vi "Lock SPAN Registers.vi"(11 "active SPAN Index":i32) -> (3 "Array":string[](array[string]))   [LabVIEW 2020, in "Linearisierung v2.lvlib" / "SpanEinstellungen.lvlib"]
uses:
  SpanEinstellungen.lvlib
  Aktion FGV SpanEinstellungen.ctl
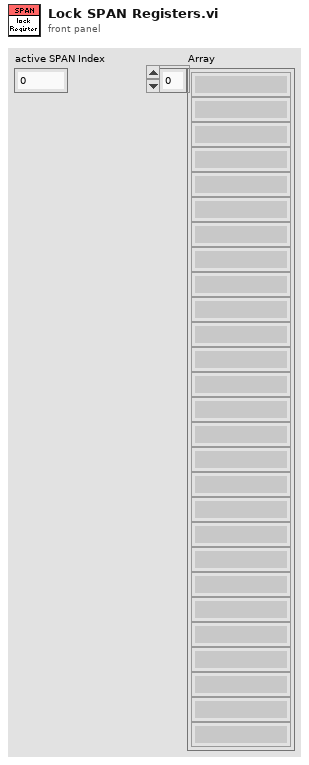
[diagram p1: front panel]
types:
  T1 = typedef "Linearisierung v2.lvlib/SpanEinstellungen.lvlib/Aktion FGV SpanEinstellungen.ctl" = enum16{"lesen", "schreiben", "laden", "speichern", "RegisterRef", "automatisch", "init", "PDF Params", "Punkte umkehren"}
  T2 = cluster{"HauptRegister in":refnum<vi>, "SpanRegister in":refnum<vi>}
  T3 = enum8{"Enabled", "Disabled", "Disabled and Grayed Out"}
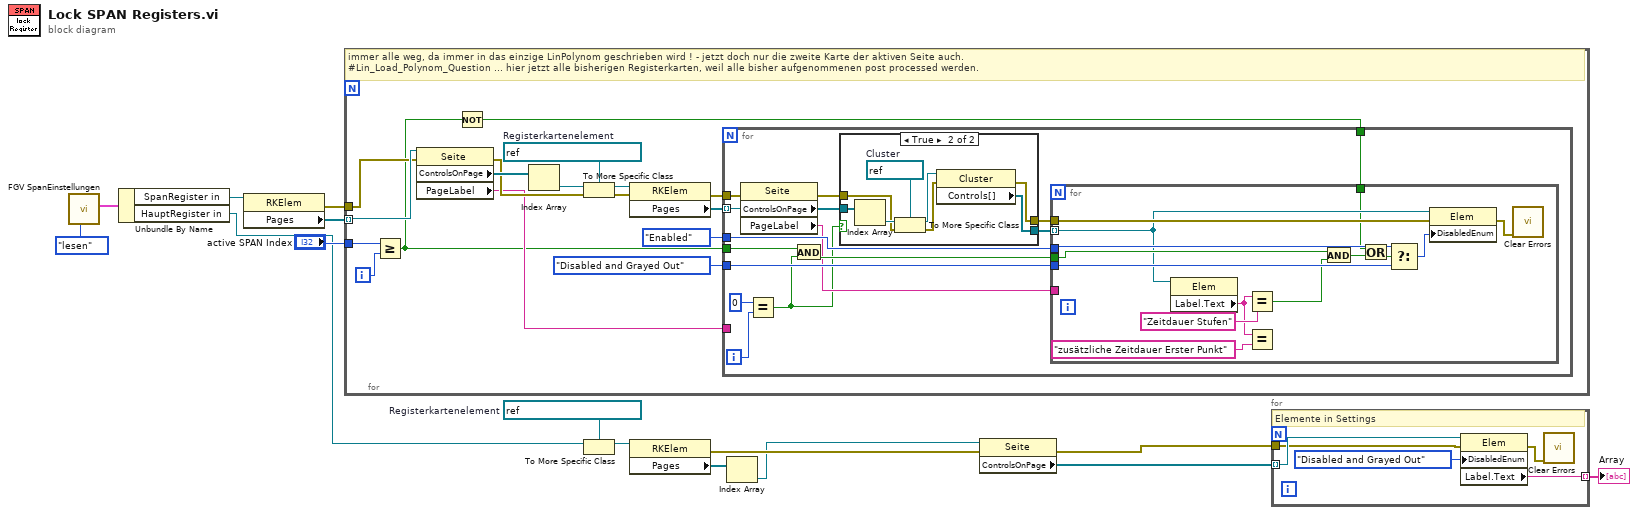
[diagram p0: block diagram]
diagram:
  w10 = refnum<vi> refnum  # Registerkartenelement
  n1 = call "FGV SpanEinstellungen.vi"("Aktion"=Aktion_FGV_SpanEinstellungen."lesen") -> ("RegisterRefs out"=w15:T2)  [unwired: 6 in, 4 out]
  n2 = Unbundle By Name(w15) -> ("SpanRegister in"=w3:refnum<vi>, "HauptRegister in"=w2:refnum<vi>)
  n3 = property class="RKElem"(reference=w3) -> (error out=w11:errorcluster, "Pages"=w12:refnum<vi>[])  [unwired: 1 in, 1 out]
  n4 = for {
    tunnel: w12 -> [w32] mode=indexing
    tunnel: w11 -> [w23]
    tunnel: "active SPAN Index" -> [w21]
    i -> [w22]
    w29 = refnum<vi> refnum  # Registerkartenelement
    # "immer alle weg, da immer in das einzige LinPolynom geschrieben wird ! - jetzt doch nur die zweite Karte der aktiven Seite auch.\n#Lin_Load_Polynom_Question ... hier jetzt alle bisherigen Registerkarten, weil alle bisher aufgenommenen post processed werden."
    n5 = Greater Or Equal?(x=w21, y=w22) -> (x >= y?=w17:bool)
    n6 = property class="Seite"(reference=w32, error in=w23) -> (error out=w26:errorcluster, "ControlsOnPage"=w31:refnum<vi>[], "PageLabel"=w20:string)  [unwired: 1 out]
    n7 = Not(x=w17) -> (.not. x?=w16:bool)
    n8 = Index Array(array=w31) -> (element=w30:refnum<vi>)  [unwired: 1 in]
    n9 = To More Specific Class(target class=w29, reference=w30, error in=w26) -> (specific class reference=w28:refnum<vi>, error out=w27:errorcluster)
    n10 = property class="RKElem"(reference=w28, error in=w27) -> (error out=w24:errorcluster, "Pages"=w25:refnum<vi>[])  [unwired: 1 out]
    n11 = for {
      tunnel: w25 -> [w47] mode=indexing
      tunnel: w24 -> [w46]
      tunnel: T3."Disabled and Grayed Out" ("Deaktiviert") -> [w42]
      tunnel: T3."Enabled" ("Deaktiviert") -> [w40]
      tunnel: w17 -> [w45]
      tunnel: w20 -> [_]
      tunnel: w16 -> [w33]
      i -> [w44]
      n12 = property class="Seite"(reference=w47, error in=w46) -> (error out=w38:errorcluster, "ControlsOnPage"=w36:refnum<vi>[], "PageLabel"=w39:string)  [unwired: 1 out]
      n13 = Equal?(x=0, y=w44) -> (x = y?=w35:bool)
      n14 = And(x=w45, y=w35) -> (x .and. y?=w41:bool)
      n15 = case shown="True" w35 {
        tunnel: w38 -> [w48 w54]
        tunnel: [w48 w57] -> w37
        tunnel: w36 -> [w49 w56]
        tunnel: [w49 w50] -> w34
        frame False {
        }
        frame True {
          w52 = refnum<vi> refnum  # Cluster
          n16 = Index Array(array=w56) -> (element=w55:refnum<vi>)  [unwired: 1 in]
          n17 = To More Specific Class(target class=w52, reference=w55, error in=w54) -> (specific class reference=w51:refnum<vi>, error out=w53:errorcluster)
          n18 = property class="Cluster"(reference=w51, error in=w53) -> (error out=w57:errorcluster, "Controls[]"=w50:refnum<vi>[])  [unwired: 1 out]
        }
      }
      n19 = for {
        tunnel: w34 -> [w64] mode=indexing
        tunnel: w37 -> [w71]
        tunnel: w42 -> [w69]
        tunnel: w41 -> [w68]
        tunnel: w40 -> [w67]
        tunnel: w39 -> [_]
        tunnel: w33 -> [w58]
        n20 = property class="Elem"(reference=w64) -> ("Label.Text"=w61:string)  [unwired: 1 in, 2 out]
        n21 = Equal?(x=w61, y="Zeitdauer Stufen") -> (x = y?=w63:bool)
        n22 = Equal?(x=w61, y="zusätzliche Zeitdauer Erster Punkt") -> ()  [unwired: 1 out]
        n23 = And(x=w68, y=w63) -> (x .and. y?=w65:bool)
        n24 = Or(x=w58, y=w65) -> (x .or. y?=w59:bool)
        n25 = Select(t=w67, s=w59, f=w69) -> (s? t:f=w66:T3)
        n26 = property class="Elem"(reference=w64, error in=w71, "DisabledEnum"=w66) -> (error out=w70:errorcluster)  [unwired: 1 out]
        n27 = call <vilib>:"Clear Errors.vi"("error in (no error)"=w70) -> ()  [unwired: 5 in, 2 out]
      }
    }
  }
  n28 = To More Specific Class(target class=w10, reference=w2) -> (specific class reference=w9:refnum<vi>)  [unwired: 1 in, 1 out]
  n29 = property class="RKElem"(reference=w9) -> (error out=w8:errorcluster, "Pages"=w7:refnum<vi>[])  [unwired: 1 in, 1 out]
  n30 = Index Array(array=w7) -> (element=w6:refnum<vi>)  [unwired: 1 in]
  n31 = property class="Seite"(reference=w6, error in=w8) -> (error out=w4:errorcluster, "ControlsOnPage"=w5:refnum<vi>[])  [unwired: 1 out]
  n32 = for {
    tunnel: w5 -> [w76] mode=indexing
    tunnel: w4 -> [w74]
    tunnel: [w72] -> w1 mode=indexing
    # "Elemente in Settings"
    n33 = property class="Elem"(reference=w76, error in=w74, "DisabledEnum"=T3."Disabled and Grayed Out" ("Deaktiviert")) -> (error out=w73:errorcluster, "Label.Text"=w72:string)  [unwired: 1 out]
    n34 = call <vilib>:"Clear Errors.vi"("error in (no error)"=w73) -> ()  [unwired: 5 in, 2 out]
  }
  "Array" <- w1
